vi "BeltControl.vi"(0 "suck in":bool, 1 "roll out":bool, 2 "Top eye":bool, 3 "Middle eye":bool, 4 "Bottom eye":bool) -> (5 "conveyerTop":dbl, 6 "conveyerMiddle":dbl, 7 "conveyerBottom":dbl)   [LabVIEW 2011]
panel:
  in  "Time Target (s)":dbl=0.1
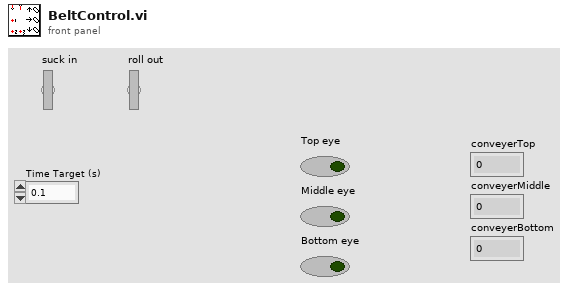
[diagram p1: front panel]
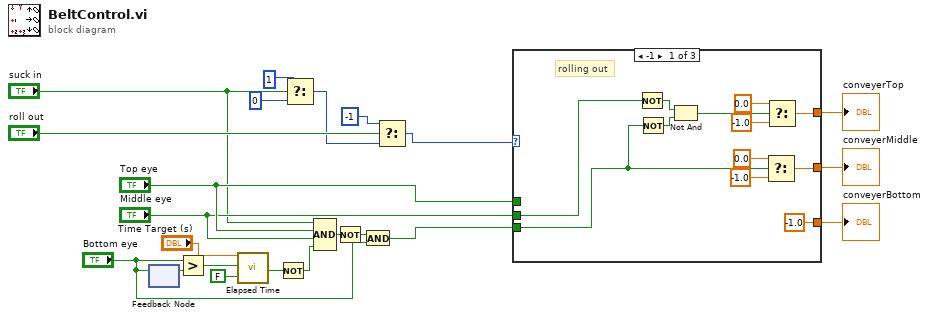
[diagram p0: block diagram]
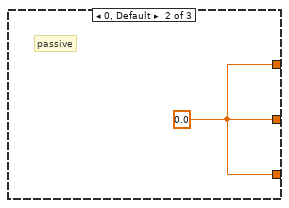
[diagram p2: hidden frame]
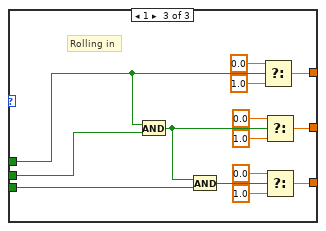
[diagram p3: hidden frame]
diagram:
  n1 = feedback-in #1("Bottom eye") -> ()
  n2 = feedback #1() -> (w12:bool)  [unwired: 1 in]
  n3 = Greater?(x="Bottom eye", y=w12) -> (0:w11:bool)
  n4 = call "Elapsed Time"("Time Target (s)"="Time Target (s)", "Reset"=w11, "Auto Reset"=FALSE) -> ("Time has Elapsed"=w10:bool)  [unwired: 9 in, 7 out]
  n5 = Not(x=w10) -> (.not. x?=w9:bool)
  n6 = Select(t=1, s="suck in", f=0) -> (s? t:f=w2:i32)
  n7 = Compound Arithmetic op=AND("suck in", "Top eye", "Middle eye", w9) -> (w6:bool)
  n8 = Not(x=w6) -> (.not. x?=w5:bool)
  n9 = And(x=w5, y="Bottom eye") -> (x .and. y?=w4:bool)
  n10 = Select(t=-1, s="roll out", f=w2) -> (s? t:f=w1:i32)
  n11 = case shown="-1" w1 {
    tunnel: "Top eye" -> [_ _ w39]
    tunnel: "Middle eye" -> [w23 _ w40]
    tunnel: w4 -> [w27 _ w38]
    tunnel: [w33 w35 w44] -> w21
    tunnel: [w28 w35 w49] -> w22
    tunnel: [-1.0 ("f") w35 w41] -> w20
    frame -1 {
      # "rolling out"
      n12 = Not(x=w23) -> (.not. x?=w26:bool)
      n13 = Not(x=w27) -> (.not. x?=w25:bool)
      n14 = Not And(1:w25, 2:w26) -> (0:w24:bool)
      n15 = Select(t=0.0, s=w27, f=-1.0) -> (s? t:f=w33:dbl)
      n16 = Select(t=0.0, s=w24, f=-1.0) -> (s? t:f=w28:dbl)
    }
    frame 0, Default {
      w35 = 0.0
      # "passive"
    }
    frame 1 {
      # "Rolling in"
      n17 = And(x=w39, y=w40) -> (x .and. y?=w36:bool)
      n18 = And(x=w36, y=w38) -> (x .and. y?=w37:bool)
      n19 = Select(t=0.0, s=w39, f=1.0) -> (s? t:f=w49:dbl)
      n20 = Select(t=0.0, s=w36, f=1.0) -> (s? t:f=w44:dbl)
      n21 = Select(t=0.0, s=w37, f=1.0) -> (s? t:f=w41:dbl)
    }
  }
  "conveyerTop" <- w22
  "conveyerMiddle" <- w21
  "conveyerBottom" <- w20
